vi "getAMtable2.vi"(11 "Serial Port Select":refnum<visa-resource-name>="COM3") -> (0 "COM Error":bool, 1 "Min dB":dbl, 2 "Max dB":dbl, 3 "Waveform Graph":dbl[](graph), 4 "AM Freq Hz":dbl, 8 "Step Delay uS":dbl)   [LabVIEW 2012]
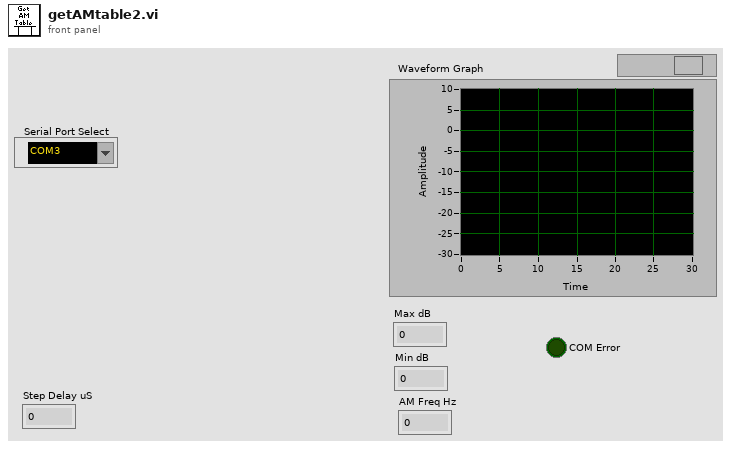
[diagram p1: front panel]
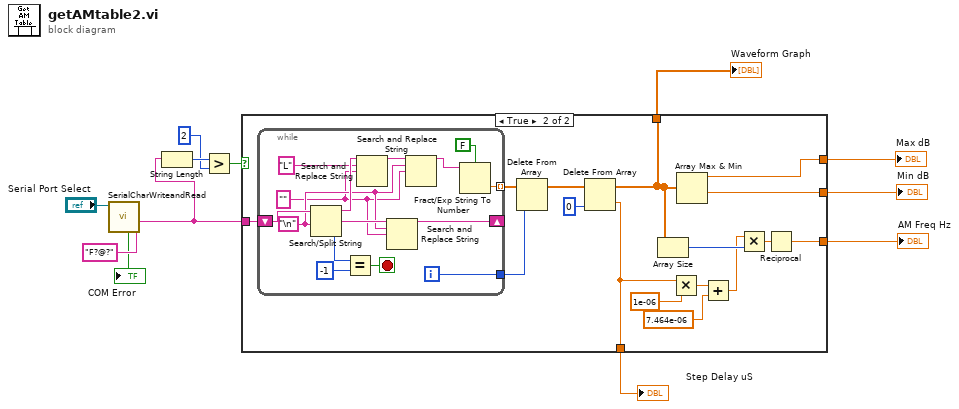
[diagram p0: block diagram]
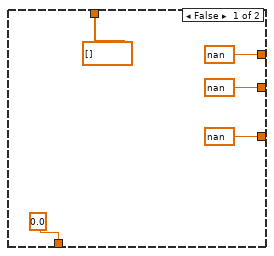
[diagram p2: hidden frame]
diagram:
  n1 = call "SerialCharWriteandRead.vi"("VISA resource name"="Serial Port Select", "write buffer"="F?@?") -> ("error?"=→"COM Error":bool, "read buffer"=w2:string)  [unwired: 5 in, 2 out]
  n2 = String Length(string=w2) -> (length=w10:i32)
  n3 = Greater?(x=w10, y=2) -> (0:w11:bool)
  n4 = case shown="True" w11 {
    tunnel: w2 -> [_ w33]
    tunnel: [dbl[] [] w19] -> w6
    tunnel: [nan w25] -> w5
    tunnel: [nan w24] -> w4
    tunnel: [nan w23] -> w3
    tunnel: [0.0 w22] -> w1
    frame False {
    }
    frame True {
      n5 = while {
        shift-right: [w40] -> _
        shift-left: w33 -> [w46]
        tunnel: [w37] -> w32
        tunnel: [w35] -> w21 mode=indexing
        i -> [w37]
        stop <- w48 stop-if-true
        w39 = "\n"
        w38 = "" ("replace string (\"\")")
        n6 = Search/Split String(string=w46, search string/char (-)=w39) -> (substring before match=w45:string, match + rest of string=w41:string, offset of match=w42:i32)  [unwired: 1 in]
        n7 = Equal?(x=w42, y=-1) -> (x = y?=w48:bool)
        n8 = Search and Replace String(input string=w45, search string="L" ("format string"), replace string=w38) -> (result string=w43:string)  [unwired: 5 in, 3 out]
        n9 = Search and Replace String(input string=w41, search string=w39, replace string=w38) -> (result string=w40:string)  [unwired: 5 in, 3 out]
        n10 = Search and Replace String(input string=w43, search string=w39, replace string=w38) -> (result string=w36:string)  [unwired: 5 in, 3 out]
        n11 = Fract/Exp String To Number(use system decimal point (T)=FALSE, string=w36) -> (number=w35:dbl)  [unwired: 2 in, 1 out]
      }
      n12 = Delete From Array(array=w21, index=w32) -> (array with subset deleted=w20:dbl[])  [unwired: 1 in, 1 out]
      n13 = Delete From Array(array=w20, index=0) -> (deleted portion=w22:dbl, array with subset deleted=w19:dbl[])  [unwired: 1 in]
      n14 = Array Size(array=w19) -> (size(s)=w31:i32)
      n15 = Multiply(x=w22, y=1e-06) -> (x*y=w28:dbl)
      n16 = Array Max & Min(array=w19) -> (max value=w25:dbl, min value=w24:dbl)  [unwired: 2 out]
      n17 = Add(x=w28, y=7.464e-06 ("x")) -> (x+y=w26:dbl)
      n18 = Multiply(x=w26, y=w31) -> (x*y=w30:dbl)
      n19 = Reciprocal(x=w30) -> (1/x=w23:dbl)
    }
  }
  "Waveform Graph" <- w6
  "Step Delay uS" <- w1
  "AM Freq Hz" <- w3
  "Min dB" <- w4
  "Max dB" <- w5
